vi "Digital Demod Trace Limit X Configure List Data.vi"(7 "ListData":dbl[](array[numeric]) format="%.2p", 8 "error in (no error)":errorcluster {"code" format="%.0x"}, 9 "ListDataBufferSize":i32=2048, 10 "DigitalDemodTraceLimit":string="TraceLimit1", 11 "instrument handle":refnum<k15>) -> (0 "error out":errorcluster {"code" format="%.0x"}, 3 "instrument handle out":refnum<k15>)   [LabVIEW 2021, in "Keysight XSAnVMA.lvlib"]
doc: "Configure a list of x values for selected limit line."
uses:
  <instrlib>/Keysight XSAnVMA/Keysight XSAnVMA.lvlib
  KtXSAnVMA_64.dll
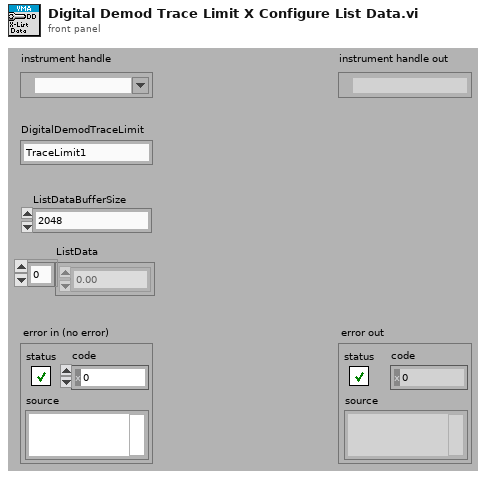
[diagram p1: front panel]
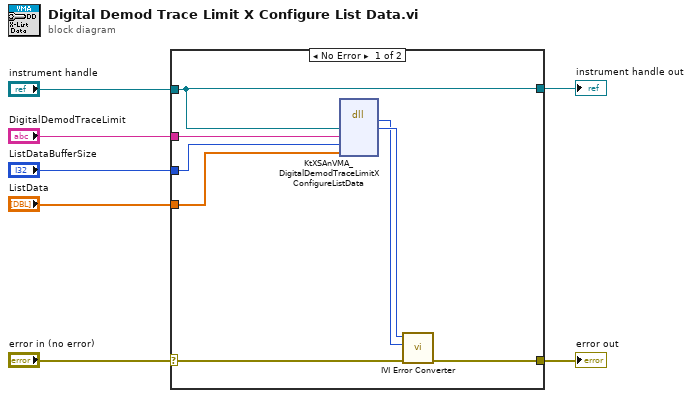
[diagram p0: block diagram]
diagram:
  n1 = case shown="No Error" "error in (no error)" {
    selector: "error in (no error)" -> [w13 w17]
    tunnel: [w12 w17] -> w7
    tunnel: "instrument handle" -> [w8 w16]
    tunnel: "DigitalDemodTraceLimit" -> [w11 _]
    tunnel: "ListDataBufferSize" -> [w10 _]
    tunnel: "ListData" -> [w9 _]
    tunnel: [w8 w16] -> w1
    frame No Error {
      n2 = dll-call lib="KtXSAnVMA**.dll" fn="KtXSAnVMA_DigitalDemodTraceLimitXConfigureListData"("Vi"=w8, "DigitalDemodTraceLimit"=w11, "ListDataBufferSize"=w10, "ListData"=w9) -> (w14:i32, "Vi"=w15:u32)  [unwired: 6 in, 2 out]
      n3 = call <instrlib>:"IVI Error Converter.vi"("error in (no error)"=w13, "IVI error code (0)"=w14, "instrument handle"=w15) -> ("error out"=w12:errorcluster)  [unwired: 7 in, 1 out]
    }
    frame Error {
    }
  }
  "error out" <- w7
  "instrument handle out" <- w1
